vi "CalculateImageSize.vi"(8 "error in (no error)":errorcluster, 10 "String":string, 11 "BarCode in":refnum<class "BarCode.lvclass">) -> (0 "error out":errorcluster, 2 "Size":cluster{"x":i16, "y":i16}, 3 "BarCode out":refnum<class "BarCode.lvclass">)   [LabVIEW 2013, in "BarCodes.lvlib" / "BarCode.lvclass"]
doc: "Calculates the size of the image for the barcode. This should include the entire barcode, quiet space, and text around it."
uses:
  BarCode.lvclass
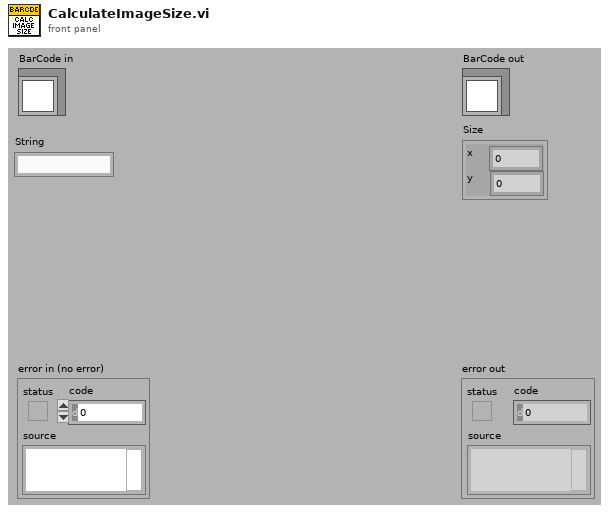
[diagram p1: front panel]
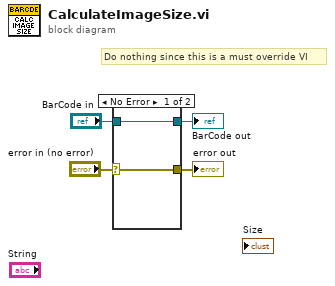
[diagram p0: block diagram]
diagram:
  # "Do nothing since this is a must override VI"
  n1 = case shown="No Error" "error in (no error)" {
    selector: "error in (no error)" -> [w5 w8]
    tunnel: [w5 w8] -> w3
    tunnel: [w6 w7] -> w1
    tunnel: "BarCode in" -> [w6 w7]
    frame No Error {
    }
    frame Error {
    }
  }
  "error out" <- w3
  "BarCode out" <- w1
